vi "Read Action.vi"(8 "error in (no error)":errorcluster, 11 "Control in":refnum<class "Control.lvclass">) -> (0 "error out":errorcluster, 2 "Action":T1 items=["Switch when pressed", "Switch when released", "Switch until release", "Latch when pressed", "Latch when released", "Latch until released"], 3 "Control out":refnum<class "Control.lvclass">)   [LabVIEW 2013, in "Control.lvclass"]
doc: "Accessor VI for the control class"
uses:
  Control.lvclass
  Typedefs/TypeDef_Action.ctl
  Control.lvclass/Control.ctl
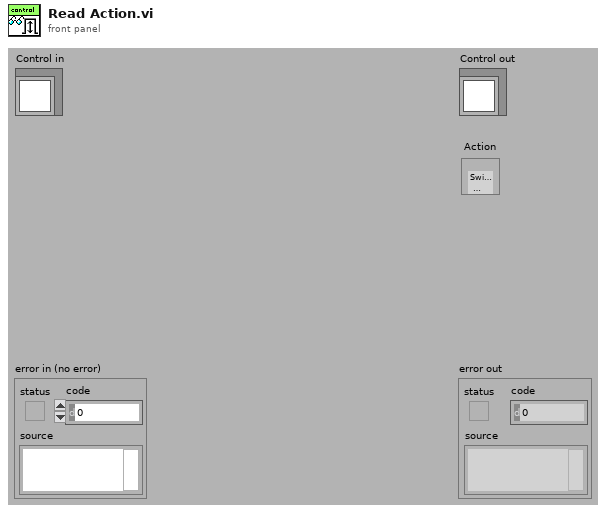
[diagram p1: front panel]
types:
  T1 = typedef "Control.lvclass/TypeDef_Action.ctl" = u16
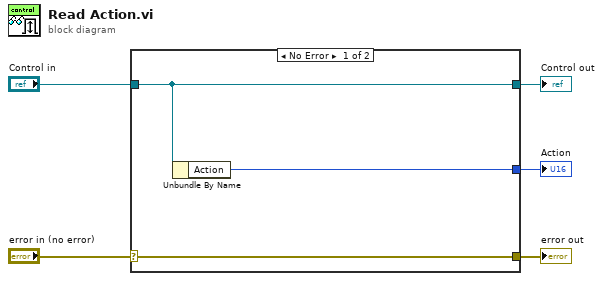
[diagram p0: block diagram]
diagram:
  n1 = case shown="No Error" "error in (no error)" {
    selector: "error in (no error)" -> [w8 w9]
    tunnel: [w8 w9] -> w4
    tunnel: [w7 w10] -> w2
    tunnel: "Control in" -> [w7 w10]
    tunnel: [w6 _] -> w1
    frame No Error {
      n2 = Unbundle By Name(w7) -> ("Action"=w6:u16)
    }
    frame Error {
    }
  }
  "error out" <- w4
  "Control out" <- w2
  "Action" <- w1
